vi "Run_VI_Named_specific.vi"(8 "Run VI Named String":string, 11 "Multi Run Row":T1 {"Row Duration (mins)" format="%#.1f"; "Row No" min=0; "Trace Gas Concentration (%)" min=0.0 format="%#.2f"; "Emission Rate (l/min)" format="%#.2f"; "Tunnel Speed" format="%#.2f"; "Start X" format="%#.2f"; "Start Y" format="%#.2f"; "Start Z" format="%#.2f"; "End X" format="%#.2f"; "End Y" format="%#.2f"; "End Z" format="%#.2f"; "Averaging time (min)" min=0.0 format="%#.2f"}) -> (0 "Scalable Time (Sec)":dbl format="%.2f", 1 "Fixed Time (Sec)":dbl format="%.2f", 2 "Channel Names":string[](array[string]), 3 "Checks":string[](array[string]), 4 "Error String":string, 5 "Check Meas Setup?":bool, 6 "Check for start NaNs?":bool)   [LabVIEW 2010]
uses:
  Gen Trav/Traverse_cluster.ctl
  Gen Trav/Spacing.ctl
  Controls/Multi_run_mode.ctl
  Globals/Preference_global.vi
panel:
  # "X           Y            Z"
  # "Start"
  # "End"
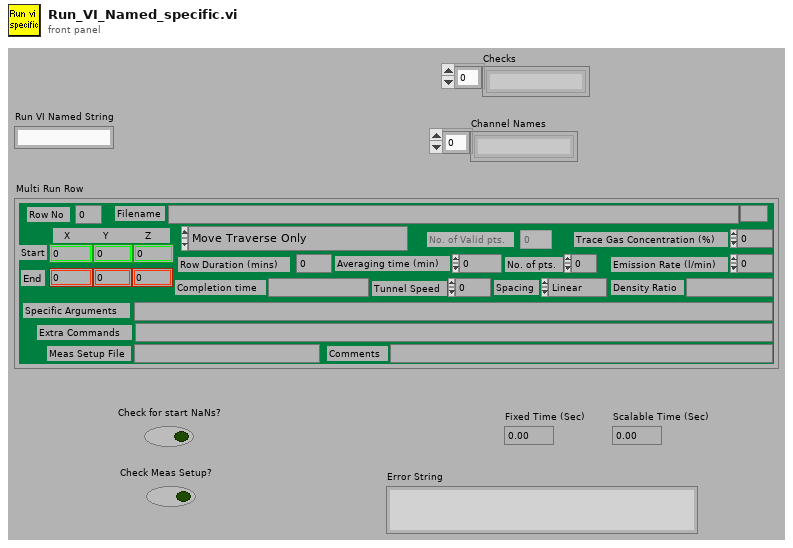
[diagram p1: front panel]
types:
  T1 = typedef "Traverse_cluster.ctl" = cluster{"Start X":dbl, "Start Y":dbl, "Start Z":dbl, "End X":dbl, "End Y":dbl, "End Z":dbl, "No. of pts.":i32, "Spacing":T2, "Filename":path, "Tunnel Speed":dbl, "Averaging time (min)":dbl, "Extra Commands":string, "Specific Arguments":string, "Emission Rate (l/min)":dbl, "Trace Gas Concentration (%)":dbl, "Density Ratio":string, "Comments":string, "Row No":i32, "Row Type Selector":T3, "Completion time":string, "Row Duration (mins)":dbl, "No. of Valid pts.":i32, "Meas Setup File":string}
  T2 = typedef "Spacing.ctl" = enum16{"Linear", "Log", "Gauss", "Specified", "N/A"}
  T3 = typedef "Multi_run_mode.ctl" = enum16{"Move Traverse Only", "Set Tunnel Speed Only", "Set Source Only", "Set Measurement Conditions", "Single Measurement", "Vertical Profile", "Lateral Profile", "Longitudinal Profile", "Explore Volume", "Multi-Axis Profile", "Auto Calibrate", "Meas Fast FID Bkgnd", "Check Beam Power", "Scanning Valve Measurement", "Run VI Named:", "Set ADAM Ch", "Wait (minutes)", "Send Message", "Synchronize With:", "Fall Back to this Row", "Turn Off Row Repeating", "Blank Row"}
  T4 = typedef "Beam_Type.ctl" = u16
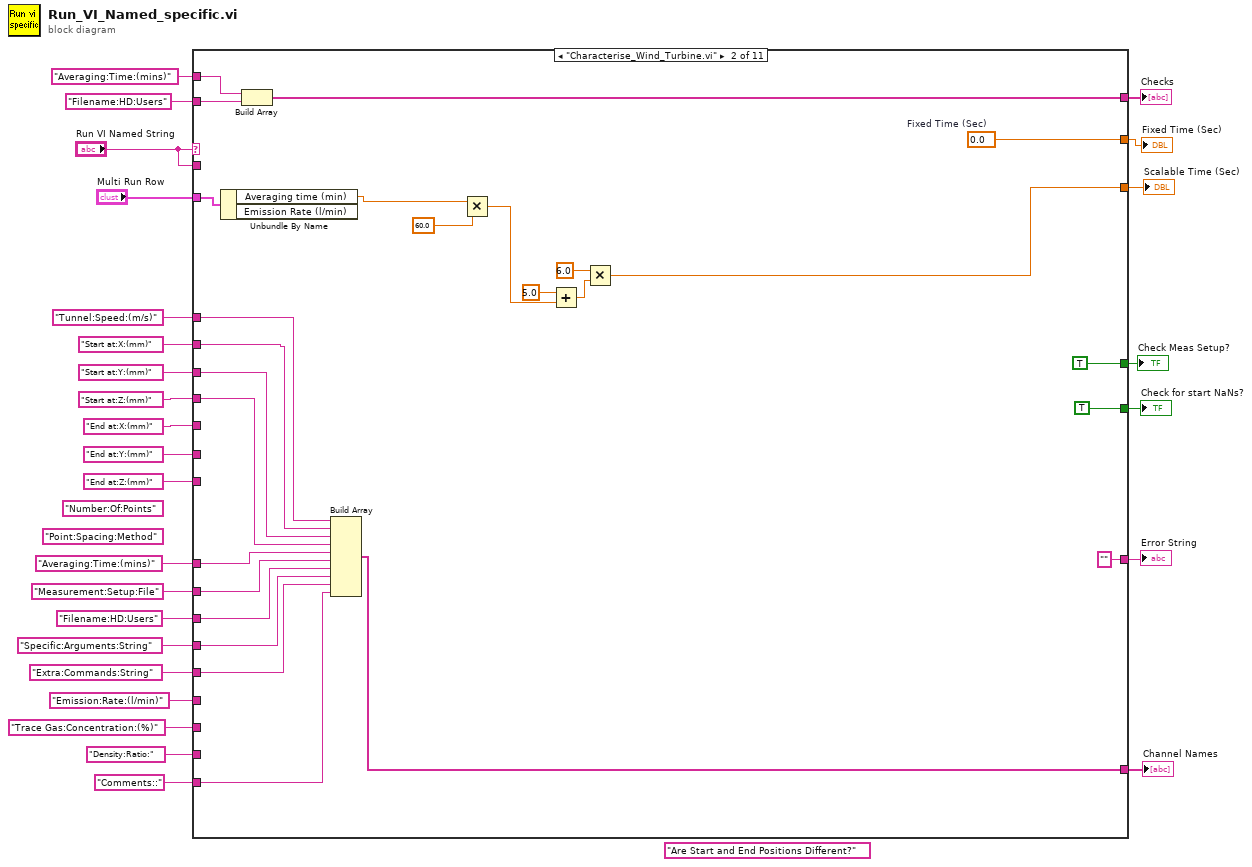
[diagram p0: block diagram]
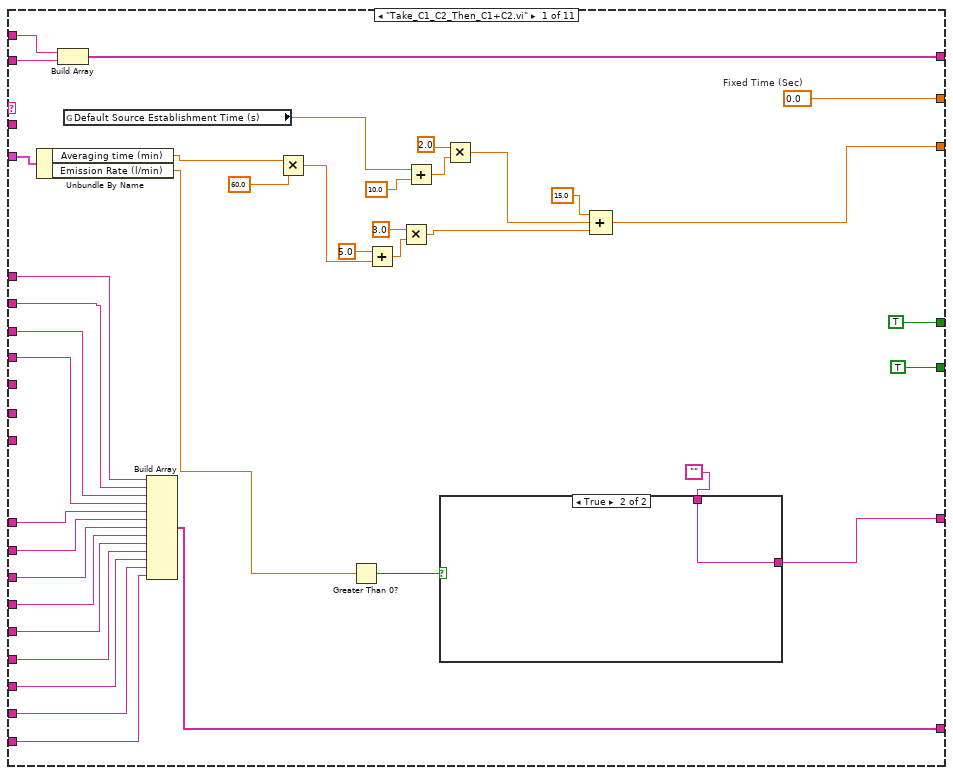
[diagram p2: hidden frame]
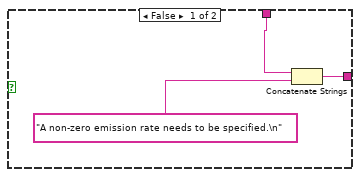
[diagram p3: hidden frame]
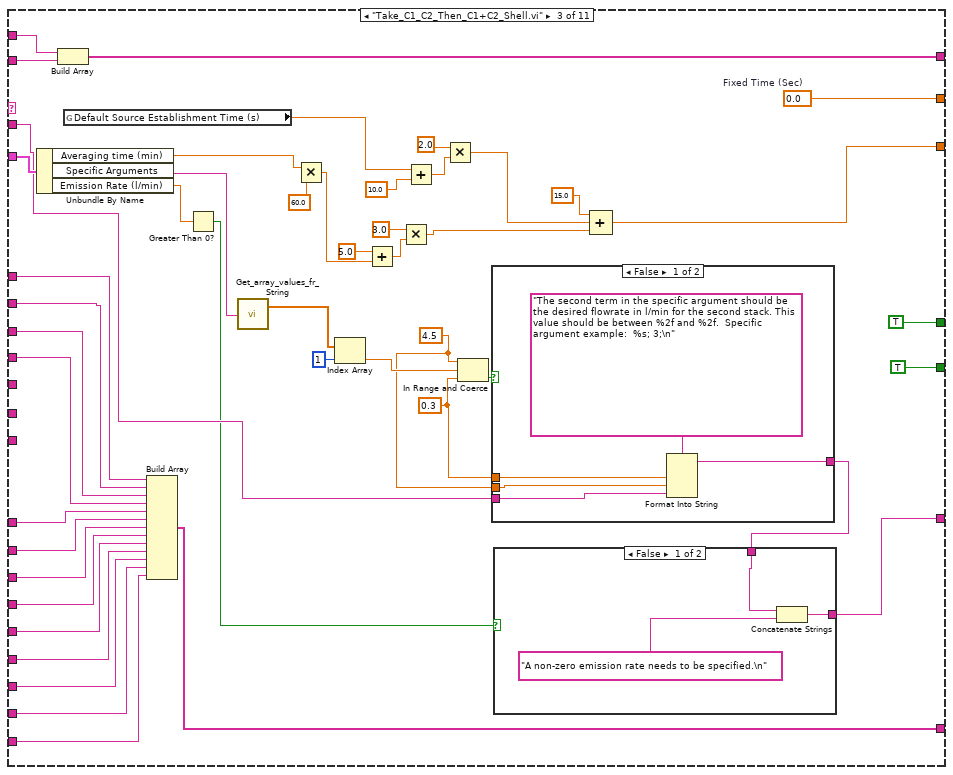
[diagram p4: hidden frame]
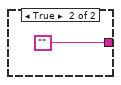
[diagram p6: hidden frame]
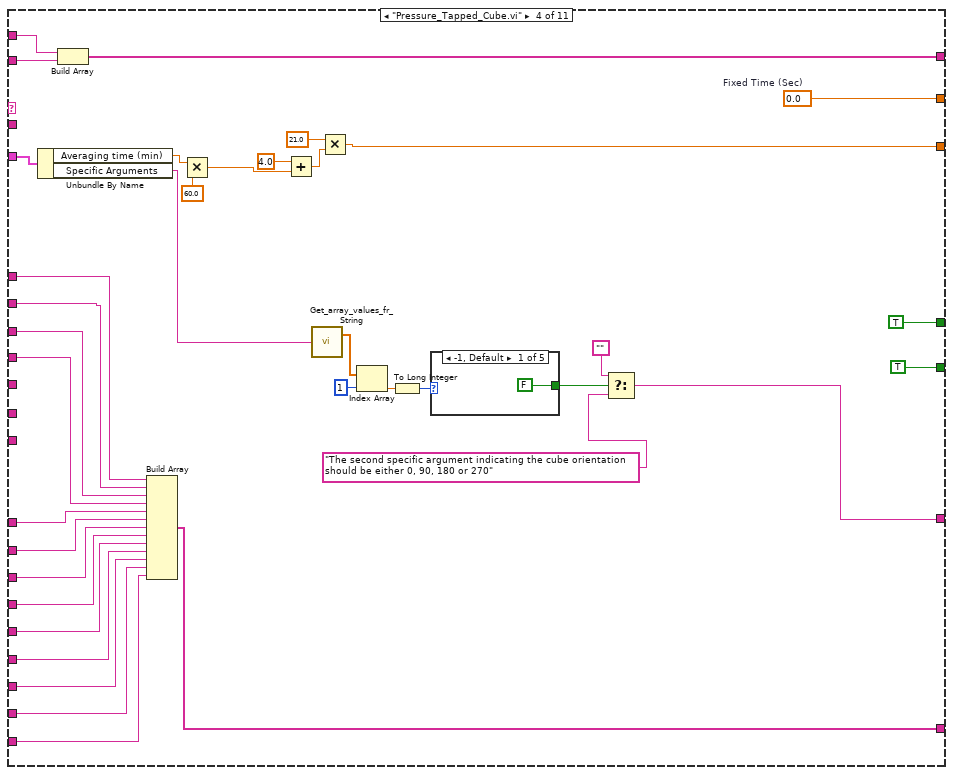
[diagram p7: hidden frame]
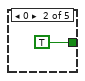
[diagram p8: hidden frame]
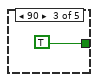
[diagram p9: hidden frame]
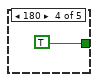
[diagram p10: hidden frame]
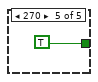
[diagram p11: hidden frame]
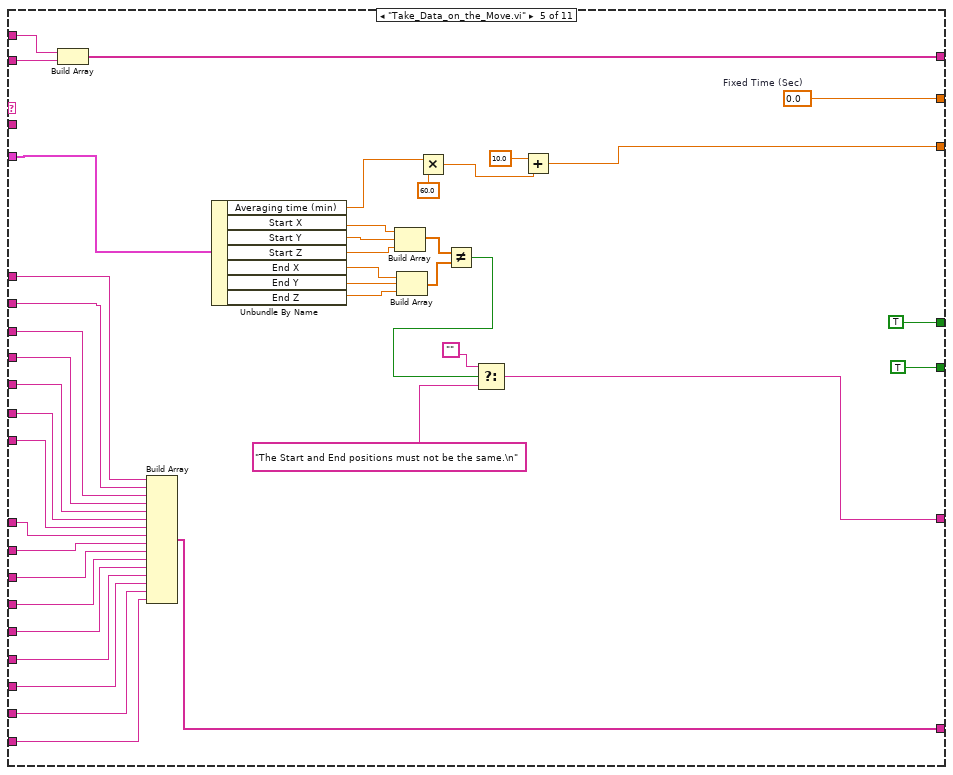
[diagram p12: hidden frame]
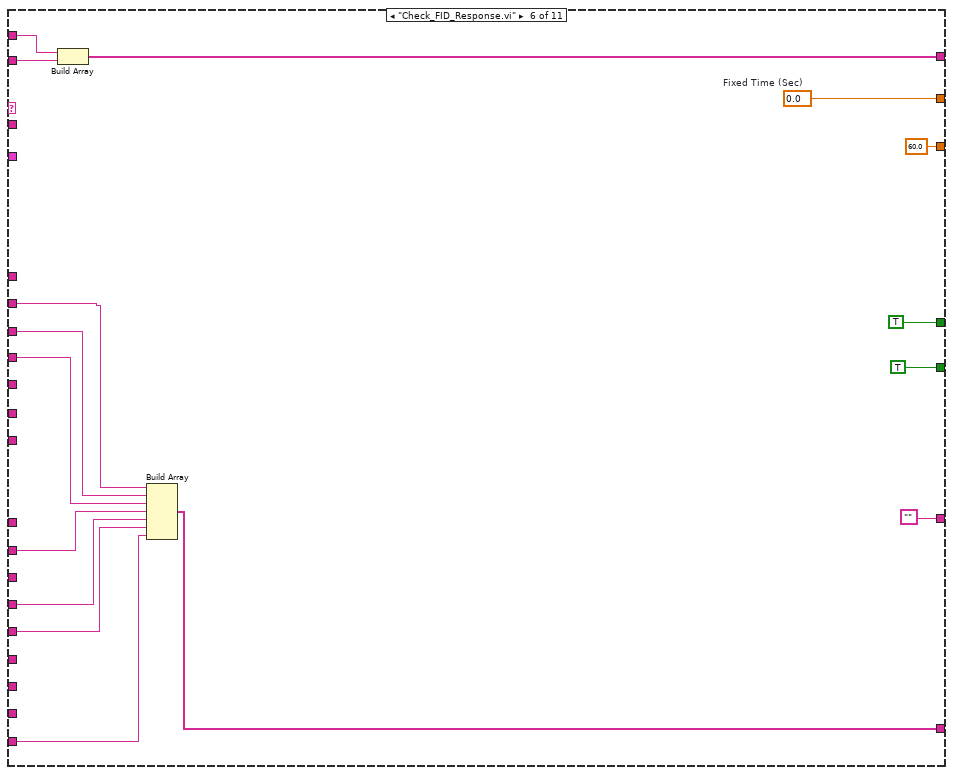
[diagram p13: hidden frame]
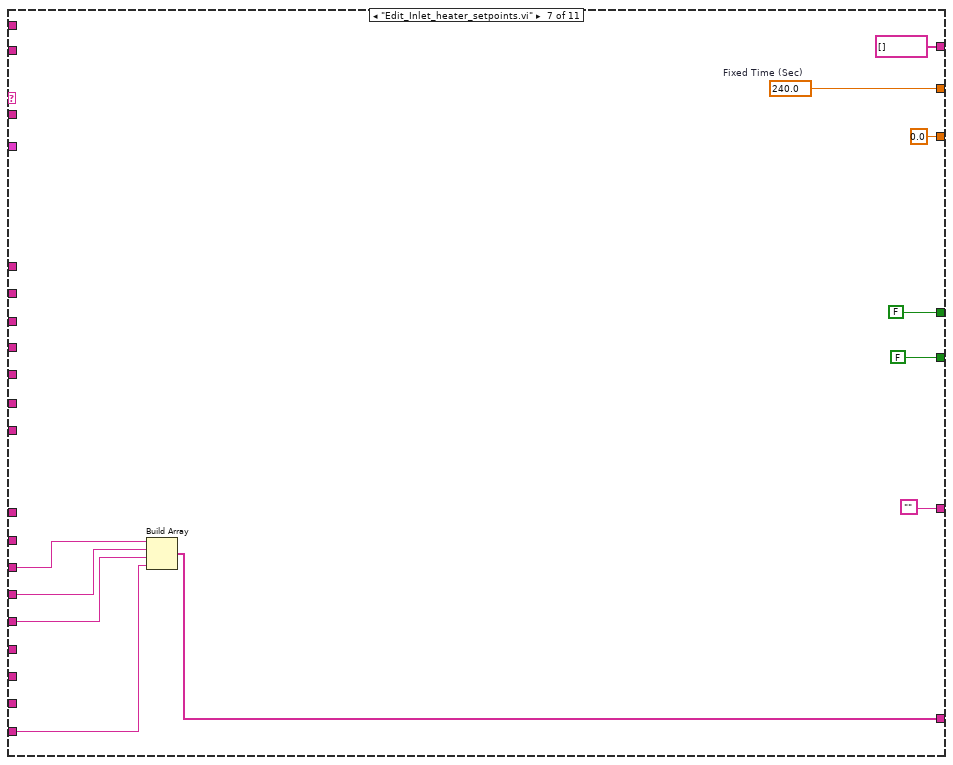
[diagram p14: hidden frame]
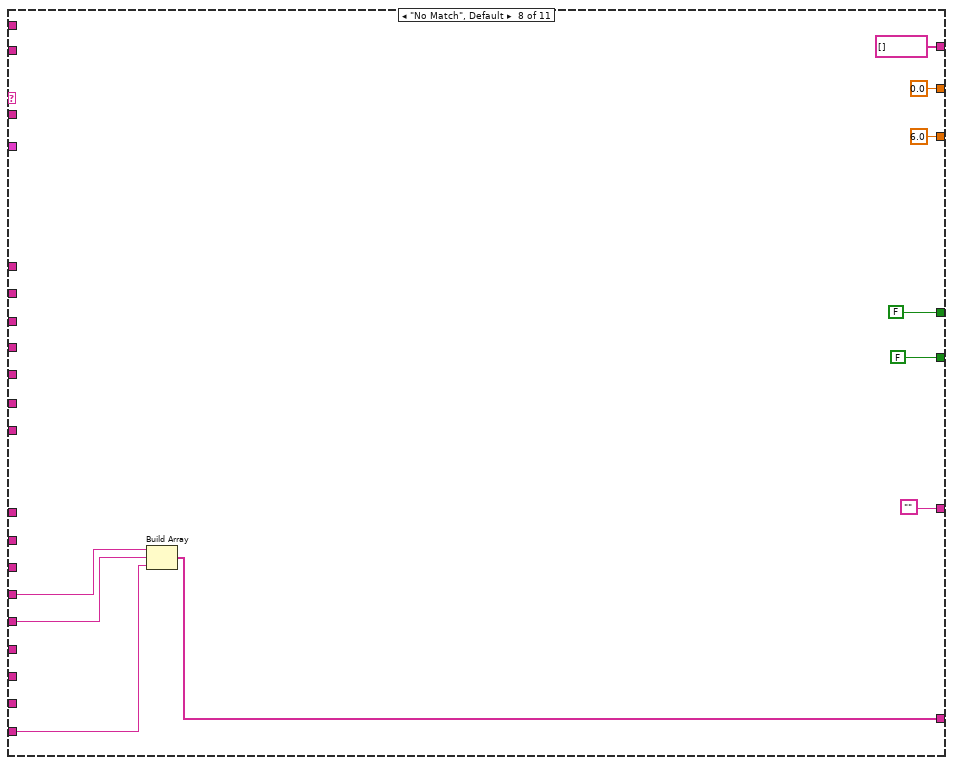
[diagram p15: hidden frame]
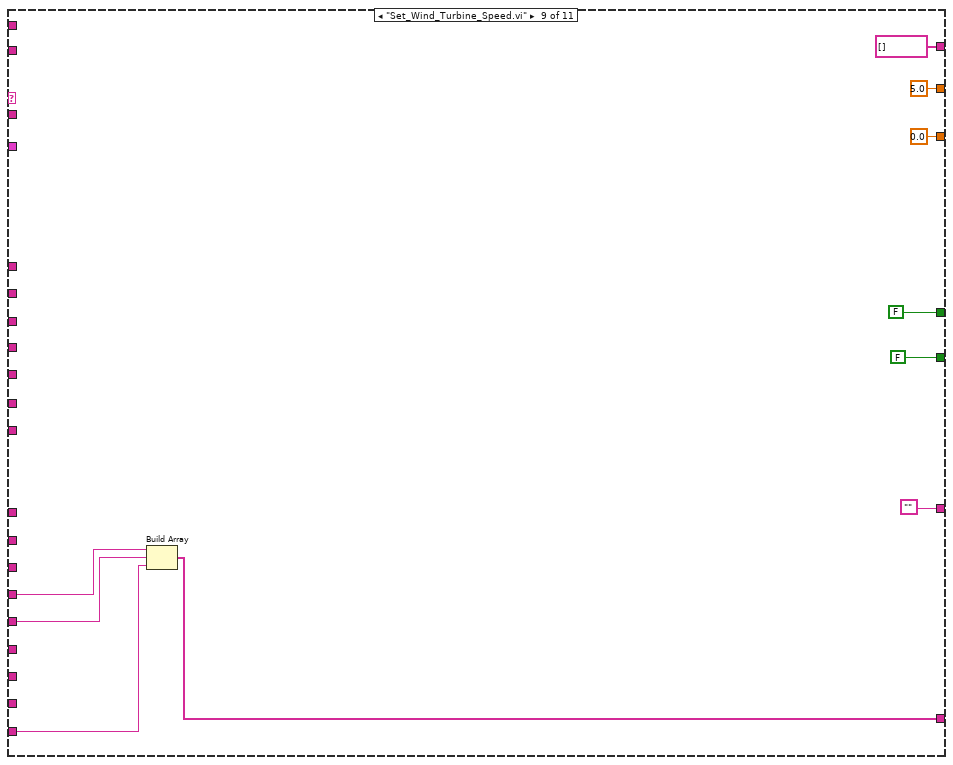
[diagram p16: hidden frame]
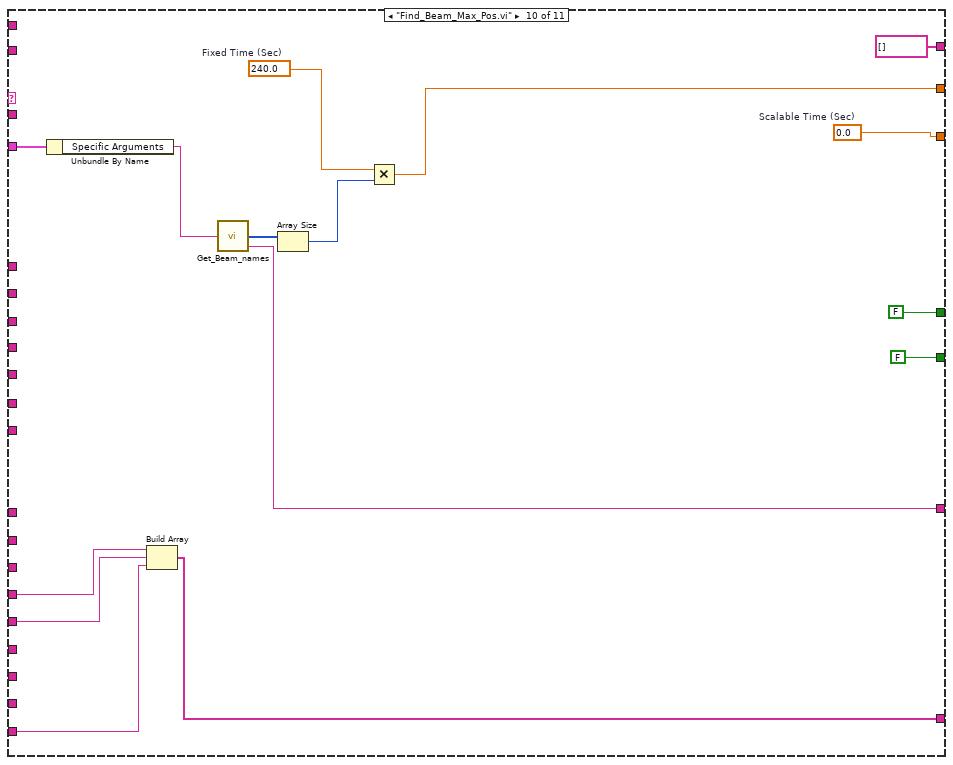
[diagram p17: hidden frame]
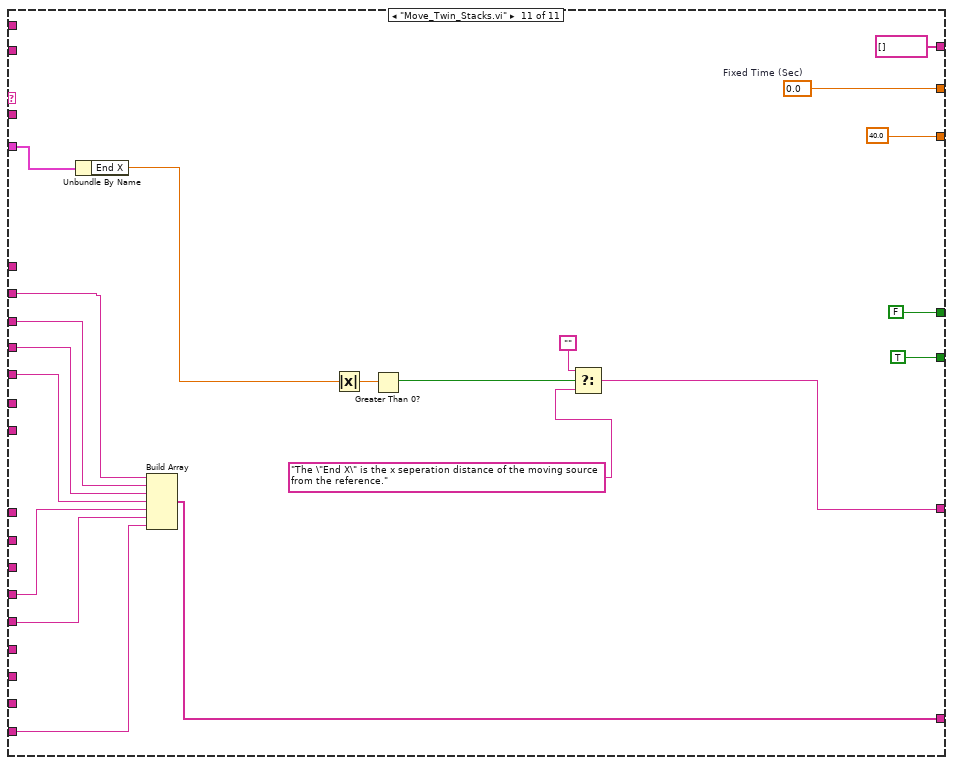
[diagram p18: hidden frame]
diagram:
  (unwired) "Point:Spacing:Method" ("Label for value")
  (unwired) "Number:Of:Points" ("Label for value")
  (unwired) "Are Start and End Positions Different?" ("Label for value")
  n1 = case shown="\"Characterise_Wind_Turbine.vi\"" "Run VI Named String" {
    tunnel: "Multi Run Row" -> [w66 w96 w143 w190 w202 _ _ _ _ w291 w318]
    tunnel: [w65 w95 w142 w189 w236 w252 w263 0.0 ("Fixed Time (Sec)") 5.0 ("Fixed Time (Sec)") w285 w317] -> w26
    tunnel: [w51 w72 w128 w163 w200 60.0 ("value") 0.0 ("value") 6.0 ("value") 0.0 ("value") w286 40.0 ("value")] -> w25
    tunnel: "Averaging:Time:(mins)" ("Label for value") -> [w50 w88 w127 w186 w234 w251 _ _ _ _ _]
    tunnel: "Filename:HD:Users" ("Label for value") -> [w49 w87 w126 w185 w233 w250 _ _ _ _ _]
    tunnel: [TRUE TRUE TRUE TRUE TRUE TRUE FALSE FALSE FALSE FALSE TRUE] -> w22
    tunnel: [TRUE TRUE TRUE TRUE TRUE TRUE FALSE FALSE FALSE FALSE FALSE] -> w21
    tunnel: [w46 w84 w123 w182 w230 w247 string[] [] string[] [] string[] [] string[] [] string[] []] -> w20
    tunnel: "Tunnel:Speed:(m/s)" ("Label for value") -> [w45 w83 w122 w181 w229 _ _ _ _ _ _]
    tunnel: "Start at:X:(mm)" ("Label for value") -> [w44 w82 w121 w180 w228 w246 _ _ _ _ w314]
    tunnel: "Start at:Y:(mm)" ("Label for value") -> [w43 w81 w120 w179 w227 w245 _ _ _ _ w313]
    tunnel: "Start at:Z:(mm)" ("Label for value") -> [w42 w80 w119 w178 w226 w244 _ _ _ _ w312]
    tunnel: "Averaging:Time:(mins)" ("Label for value") -> [w41 w79 w118 w177 w225 _ _ _ _ _ _]
    tunnel: "Measurement:Setup:File" ("Label for value") -> [w40 w78 w117 w176 w224 w243 _ _ _ _ _]
    tunnel: "Filename:HD:Users" ("Label for value") -> [w39 w77 w116 w175 w223 _ w253 _ _ _ _]
    tunnel: "Specific:Arguments:String" ("Label for value") -> [w38 w76 w115 w174 w222 w242 w260 w271 w281 w296 w300]
    tunnel: "Extra:Commands:String" ("Label for value") -> [w37 w75 w114 w173 w221 w241 w259 w270 w280 w295 w299]
    tunnel: "Emission:Rate:(l/min)" ("Label for value") -> [w36 _ w113 w172 w220 _ _ _ _ _ _]
    tunnel: "Trace Gas:Concentration:(%)" ("Label for value") -> [w35 _ w112 w171 w219 _ _ _ _ _ _]
    tunnel: "Density:Ratio:" ("Label for value") -> [w34 _ w111 w170 w218 _ _ _ _ _ _]
    tunnel: "Comments::" ("Label for value") -> [w33 w74 w110 w169 w217 w240 w258 w269 w279 w294 w308]
    tunnel: [w32 w73 w109 w168 w216 w239 w257 w268 w278 w293 w311] -> w6
    tunnel: [w30 "" ("Error Comments") w97 w154 w199 "" "" "" "" w284 w302] -> w5
    tunnel: "End at:X:(mm)" ("Label for value") -> [_ _ _ _ w198 _ _ _ _ _ w309]
    tunnel: "End at:Y:(mm)" ("Label for value") -> [_ _ _ _ w197 _ _ _ _ _ _]
    tunnel: "End at:Z:(mm)" ("Label for value") -> [_ _ _ _ w196 _ _ _ _ _ _]
    tunnel: "Run VI Named String" -> [_ _ w103 _ _ _ _ _ _ _ _]
    frame "Take_C1_C2_Then_C1+C2.vi" {
      w65 = 0.0  # Fixed Time (Sec)
      n2 = Unbundle By Name(w66) -> ("Averaging time (min)"=w54:dbl, "Emission Rate (l/min)"=w29:dbl)
      n3 = Build Array(w50, w49) -> (w46:string[])
      n4 = global read "Preference_global.vi" "Default Source Establishment Time (s)"() -> (w55:dbl)
      n5 = Build Array(w45, w44, w43, w42, w41, w40, w39, w38, w37, w36, w35, w34, w33) -> (w32:string[])
      n6 = Multiply(x=w54, y=60.0) -> (x*y=w52:dbl)
      n7 = Greater Than 0?(x=w29) -> (x > 0?=w28:bool)
      n8 = Add(x=5.0, y=w52) -> (x+y=w58:dbl)
      n9 = Multiply(x=3.0, y=w58) -> (x*y=w62:dbl)
      n10 = Add(x=w55, y=10.0) -> (x+y=w60:dbl)
      n11 = case shown="True" w28 {
        tunnel: "" -> [w68 w70]
        tunnel: [w67 w70] -> w30
        frame False {
          n12 = Concatenate Strings(w68, "A non-zero emission rate needs to be specified.\n") -> (w67:string)
        }
        frame True {
        }
      }
      n13 = Multiply(x=2.0, y=w60) -> (x*y=w63:dbl)
      n14 = Compound Arithmetic op=ADD(15.0 ("value"), w63, w62) -> (w51:dbl)
    }
    frame "Characterise_Wind_Turbine.vi" {
      w95 = 0.0  # Fixed Time (Sec)
      n15 = Unbundle By Name(w96) -> ("Averaging time (min)"=w91:dbl)  [unwired: 1 out]
      n16 = Build Array(w88, w87) -> (w84:string[])
      n17 = Build Array(w83, w82, w81, w80, w79, w78, w77, w76, w75, w74) -> (w73:string[])
      n18 = Multiply(x=w91, y=60.0) -> (x*y=w89:dbl)
      n19 = Add(x=5.0, y=w89) -> (x+y=w94:dbl)
      n20 = Multiply(x=6.0, y=w94) -> (x*y=w72:dbl)
    }
    frame "Take_C1_C2_Then_C1+C2_Shell.vi" {
      w101 = 4.5 ("upper limit")
      w102 = 0.3 ("lower limit")
      w142 = 0.0  # Fixed Time (Sec)
      n21 = Unbundle By Name(w143) -> ("Averaging time (min)"=w131:dbl, "Specific Arguments"=w106:string, "Emission Rate (l/min)"=w100:dbl)
      n22 = Build Array(w127, w126) -> (w123:string[])
      n23 = global read "Preference_global.vi" "Default Source Establishment Time (s)"() -> (w132:dbl)
      n24 = Build Array(w122, w121, w120, w119, w118, w117, w116, w115, w114, w113, w112, w111, w110) -> (w109:string[])
      n25 = Greater Than 0?(x=w100) -> (x > 0?=w99:bool)
      n26 = call "Get_array_values_fr_String.vi"("String Value"=w106) -> ("Numeric Array"=w108:dbl[])  [unwired: 1 out]
      n27 = Multiply(x=w131, y=60.0) -> (x*y=w129:dbl)
      n28 = Index Array(array=w108, index=1) -> (element=w105:dbl)
      n29 = Add(x=5.0, y=w129) -> (x+y=w135:dbl)
      n30 = Multiply(x=3.0, y=w135) -> (x*y=w139:dbl)
      n31 = Add(x=w132, y=10.0) -> (x+y=w137:dbl)
      n32 = Multiply(x=2.0, y=w137) -> (x*y=w140:dbl)
      n33 = In Range and Coerce(upper limit=w101, x=w105, lower limit=w102) -> (In Range?=w104:bool)  [unwired: 1 out]
      n34 = case shown="False" w104 {
        tunnel: [w148 ""] -> w98
        tunnel: w103 -> [w152 _]
        tunnel: w102 -> [w151 _]
        tunnel: w101 -> [w150 _]
        frame False {
          n35 = Format Into String(format string="The second term in the specific argument should be the desired flowrate in l/min for the second stack. This value should be between %2f and %2f.  Specific argument example:  %s; 3;\n", w151, w150, w152) -> (resulting string=w148:string)  [unwired: 2 in, 1 out]
        }
        frame True {
        }
      }
      n36 = case shown="False" w99 {
        tunnel: w98 -> [w145 w147]
        tunnel: [w144 w147] -> w97
        frame False {
          n37 = Concatenate Strings(w145, "A non-zero emission rate needs to be specified.\n") -> (w144:string)
        }
        frame True {
        }
      }
      n38 = Compound Arithmetic op=ADD(15.0 ("value"), w140, w139) -> (w128:dbl)
    }
    frame "Pressure_Tapped_Cube.vi" {
      w189 = 0.0  # Fixed Time (Sec)
      n39 = Unbundle By Name(w190) -> ("Averaging time (min)"=w188:dbl, "Specific Arguments"=w155:string)
      n40 = Build Array(w186, w185) -> (w182:string[])
      n41 = Build Array(w181, w180, w179, w178, w177, w176, w175, w174, w173, w172, w171, w170, w169) -> (w168:string[])
      n42 = Multiply(x=w188, y=60.0) -> (x*y=w164:dbl)
      n43 = Add(x=4.0, y=w164) -> (x+y=w167:dbl)
      n44 = call "Get_array_values_fr_String.vi"("String Value"=w155) -> ("Numeric Array"=w157:dbl[])  [unwired: 1 out]
      n45 = Multiply(x=21.0, y=w167) -> (x*y=w163:dbl)
      n46 = Index Array(array=w157, index=1) -> (element=w158:dbl)
      n47 = To Long Integer(number=w158) -> (32bit integer=w159:i32)
      n48 = case shown="-1, Default" w159 {
        tunnel: [FALSE TRUE TRUE TRUE TRUE] -> w162
        frame -1, Default {
        }
        frame 0 {
        }
        frame 90 {
        }
        frame 180 {
        }
        frame 270 {
        }
      }
      n49 = Select(t="", s=w162, f="The second specific argument indicating the cube orientation should be either 0, 90, 180 or 270") -> (s? t:f=w154:string)
    }
    frame "Take_Data_on_the_Move.vi" {
      w236 = 0.0  # Fixed Time (Sec)
      n50 = Build Array(w234, w233) -> (w230:string[])
      n51 = Build Array(w229, w228, w227, w226, w198, w197, w196, w225, w224, w223, w222, w221, w220, w219, w218, w217) -> (w216:string[])
      n52 = Unbundle By Name(w202) -> ("Averaging time (min)"=w201:dbl, "Start X"=w203:dbl, "Start Y"=w204:dbl, "Start Z"=w205:dbl, "End X"=w206:dbl, "End Y"=w207:dbl, "End Z"=w208:dbl)
      n53 = Build Array(w203, w204, w205) -> (w210:dbl[])
      n54 = Build Array(w206, w207, w208) -> (w209:dbl[])
      n55 = Multiply(x=w201, y=60.0) -> (x*y=w214:dbl)
      n56 = Not Equal?(x=w210, y=w209) -> (x != y?=w213:bool)
      n57 = Select(t="", s=w213, f="The Start and End positions must not be the same.\n" ("Format String")) -> (s? t:f=w199:string)
      n58 = Add(x=10.0, y=w214) -> (x+y=w200:dbl)
    }
    frame "Check_FID_Response.vi" {
      w252 = 0.0  # Fixed Time (Sec)
      n59 = Build Array(w251, w250) -> (w247:string[])
      n60 = Build Array(w246, w245, w244, w243, w242, w241, w240) -> (w239:string[])
    }
    frame "Edit_Inlet_heater_setpoints.vi" {
      w263 = 240.0  # Fixed Time (Sec)
      n61 = Build Array(w253, w260, w259, w258) -> (w257:string[])
    }
    frame "No Match", Default {
      n62 = Build Array(w271, w270, w269) -> (w268:string[])
    }
    frame "Set_Wind_Turbine_Speed.vi" {
      n63 = Build Array(w281, w280, w279) -> (w278:string[])
    }
    frame "Find_Beam_Max_Pos.vi" {
      w290 = 240.0  # Fixed Time (Sec)
      w286 = 0.0  # Scalable Time (Sec)
      n64 = Unbundle By Name(w291) -> ("Specific Arguments"=w287:string)
      n65 = Build Array(w296, w295, w294) -> (w293:string[])
      n66 = call "Get_Beam_names.vi"("String Value"=w287) -> ("Beam Array"=w288:T4[], "Error Comments"=w284:string)  [unwired: 1 out]
      n67 = Array Size(array=w288) -> (size(s)=w289:i32)
      n68 = Multiply(x=w290, y=w289) -> (x*y=w285:dbl)
    }
    frame "Move_Twin_Stacks.vi" {
      w317 = 0.0  # Fixed Time (Sec)
      n69 = Unbundle By Name(w318) -> ("End X"=w305:dbl)
      n70 = Build Array(w314, w313, w312, w309, w300, w299, w308) -> (w311:string[])
      n71 = Absolute Value(x=w305) -> (abs(x)=w304:dbl)
      n72 = Greater Than 0?(x=w304) -> (x > 0?=w307:bool)
      n73 = Select(t="", s=w307, f="The \"End X\" is the x seperation distance of the moving source from the reference.") -> (s? t:f=w302:string)
    }
  }
  "Fixed Time (Sec)" <- w26
  "Scalable Time (Sec)" <- w25
  "Check Meas Setup?" <- w21
  "Error String" <- w5
  "Check for start NaNs?" <- w22
  "Checks" <- w20
  "Channel Names" <- w6
